vi "Serialize Core.vi"(8 "error in (no error)":errorcluster, 11 "Serializable Message in":refnum<class "Display Text Msg.lvclass">) -> (0 "error out":errorcluster, 2 "Serialized Message":string)   [LabVIEW 2020, in "Chat Window.lvlib" / "Display Text Msg.lvclass"]
uses:
  Display Text Msg.lvclass
  Display Text Msg.lvclass/Display Text Msg.ctl
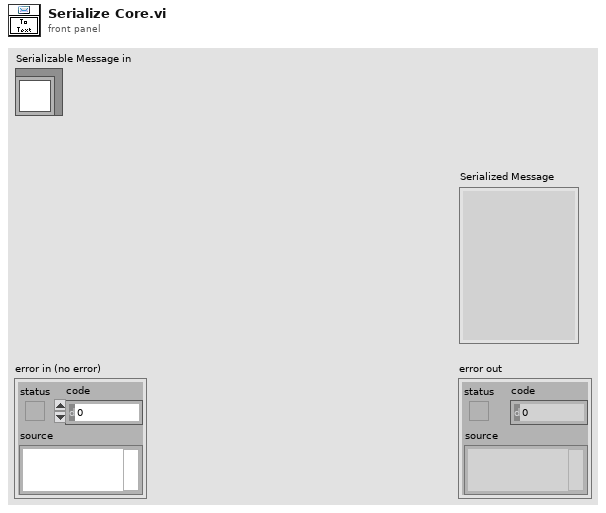
[diagram p1: front panel]
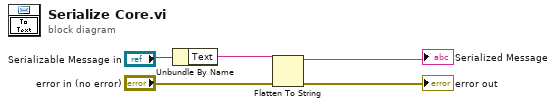
[diagram p0: block diagram]
diagram:
  n1 = Unbundle By Name("Serializable Message in") -> ("Text"=w4:string)
  n2 = Flatten To String(anything=w4, error in (no error)="error in (no error)") -> (data string=→"Serialized Message":string, error out=→"error out":errorcluster)  [unwired: 2 in, 1 out]
